vi "VS-Temp Calibration.vi"(0 "Scale":T1={"Slope"=0.0, "Offset"=0.0, "Limits"={"Min"=0.0, "Max"=0.0}, "term config"=-1} {"term config" items=["default"=-1, "RSE"=10083, "NRSE"=10078, "Differential"=10106, "Pseudodifferential"=12529]}) -> (4 "Cluster out":T1={"Slope"=0.0, "Offset"=0.0, "Limits"={"Min"=0.0, "Max"=0.0}, "term config"=-1} {"term config" items=["default"=-1, "RSE"=10083, "NRSE"=10078, "Differential"=10106, "Pseudodifferential"=12529]}, 8 "Canceled?":bool)   [LabVIEW 2020]
uses:
  Typedefs/PhysMon-Scale.ctl
  epl-vi-lib/Utility VIs/Array Manipulation VIs/Sort and Index (DBL).vi
  <vilib>/Analysis/NI_AALPro.lvlib
panel:
  out "Temp Offset In":dbl caption="Offset (deg C)"
  out "Temp Slope In":dbl caption="Scale (deg C/V)"
  in  "Temp Offset":dbl caption="Offset (deg C)"
  in  "Temp Slope":dbl caption="Scale (deg C/V)"
  in  "Fit line":bool
  out "Table":string[][](table)
  in  "Measure":bool
  in  "Temp (C)":dbl
  out "XY Graph":cluster{dbl[], dbl[]}[](graph)
  in  "Cancel":bool
  in  "OK":bool
  # "Previous"
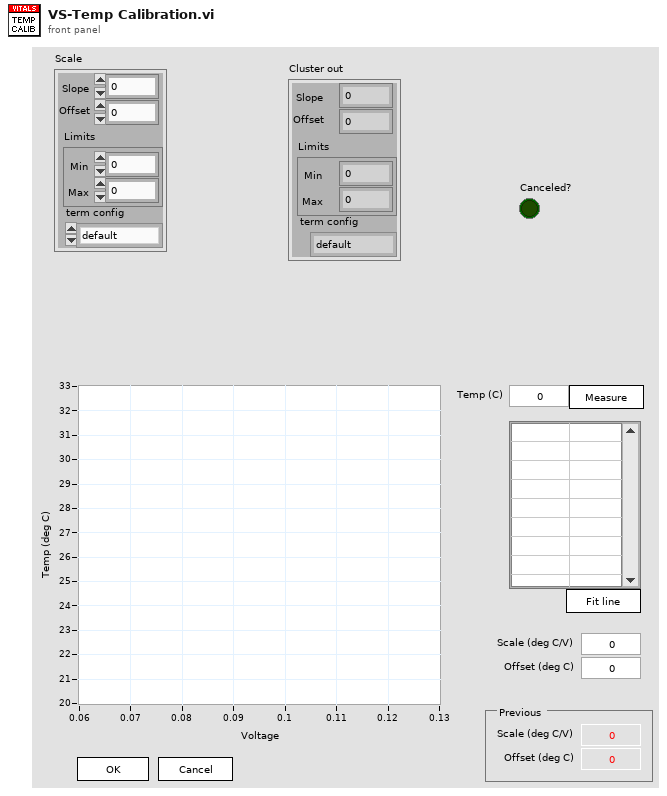
[diagram p1: front panel]
types:
  T1 = typedef "PhysMon-Scale.ctl" = cluster{"Slope":dbl, "Offset":dbl, "Limits":cluster{"Min":dbl, "Max":dbl}, "term config":i32}
  T2 = enum8{"Enabled", "Disabled", "Disabled and Grayed Out"}
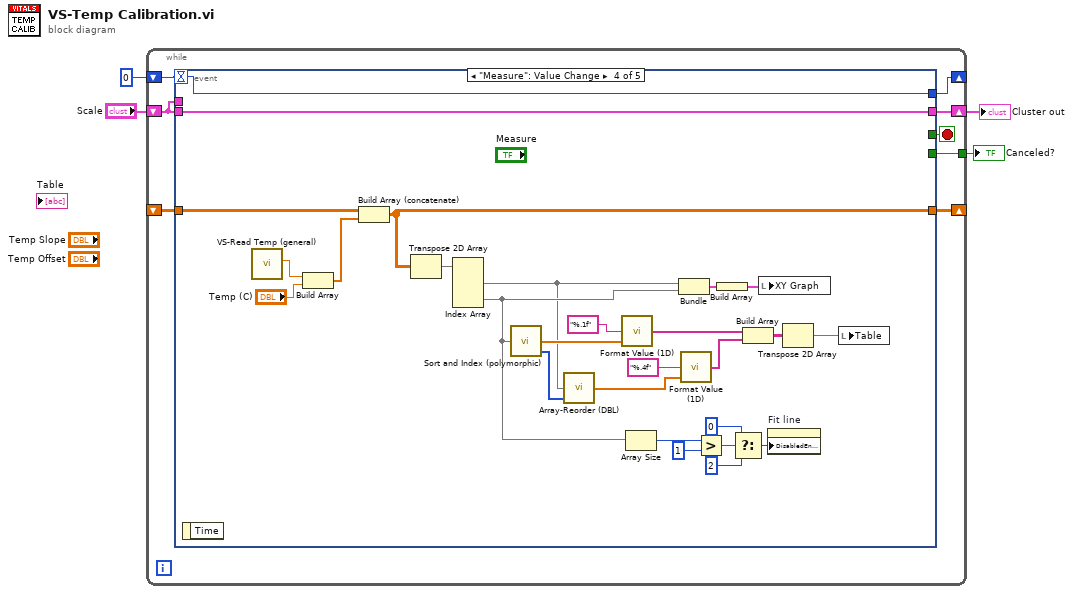
[diagram p0: block diagram]
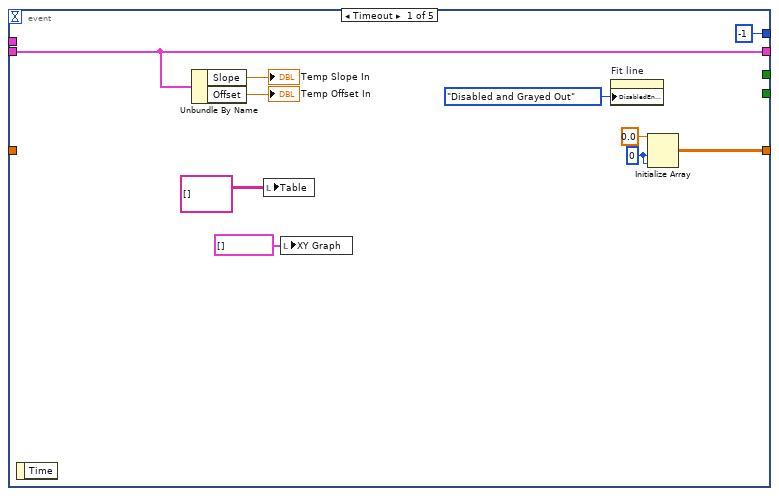
[diagram p2: hidden frame]
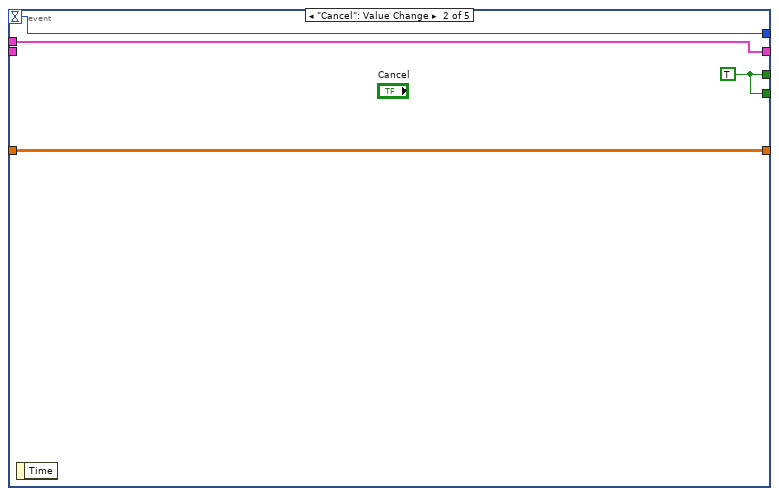
[diagram p3: hidden frame]
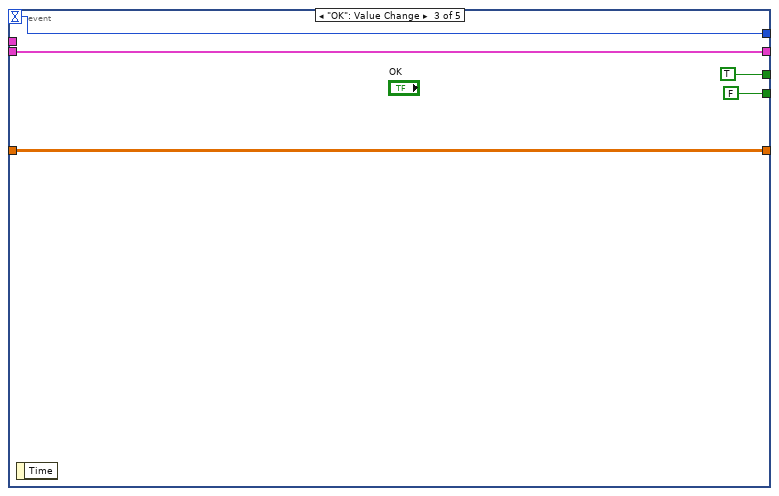
[diagram p4: hidden frame]
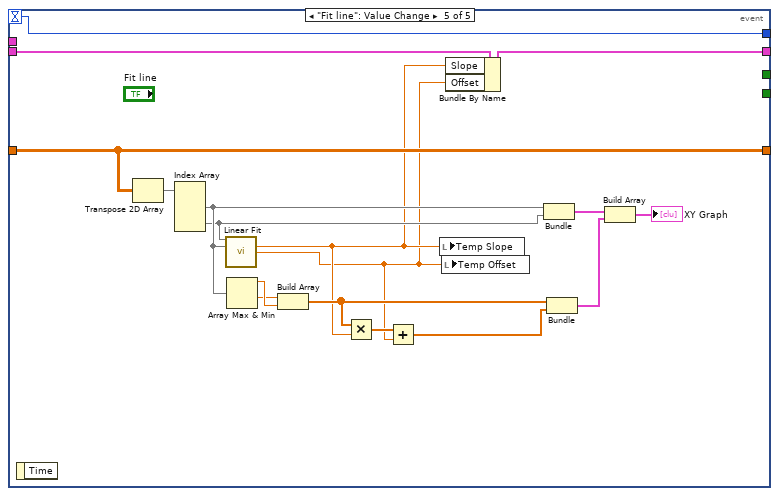
[diagram p5: hidden frame]
diagram:
  n1 = while {
    shift-right: [w11] -> _
    shift-left: 0 -> [w12]
    tunnel: [w8] -> w1
    shift-right: [w10] -> w2
    shift-left: "Scale" -> [w7]
    shift-right: [w6] -> _
    shift-left: _ -> [w5]
    stop <- w9 stop-if-true
    n2 = event shown="[3] \"Measure\": Value Change" {
      selector: _ -> [_ _ _ _ _]
      dyn-events: _ -> [_ _ _ _ _]
      timeout: w12 -> [_ w26 w30 w58 w75]
      tunnel: [-1 w26 w30 w58 w75] -> w11
      tunnel: w7 -> [w21 _ w31 w57 w74]
      tunnel: [w21 w24 w31 w57 w61] -> w10
      tunnel: [_ w25 TRUE _ _] -> w9
      tunnel: [_ w25 FALSE _ _] -> w8
      tunnel: w7 -> [_ w24 _ _ _]
      tunnel: [w16 w23 w27 w53 w73] -> w6
      tunnel: w5 -> [_ w23 w27 w56 w73]
      event Timeout {
        w15 = 0 ("dimension size")
        n3 = event-data() -> ()  [unwired: 1 in, 1 out]
        n4 = Unbundle By Name(w21) -> ("Slope"=→"Temp Slope In":dbl, "Offset"=→"Temp Offset In":dbl)
        n5 = local write "Table"(string[][] [] ("Table Control")) -> ()
        n6 = local write "XY Graph"(cluster{dbl[], dbl[]}[] [] ("XY Graph")) -> ()
        n7 = property on="Fit line" class="Bool"("DisabledEnum"=T2."Disabled and Grayed Out" ("Disabled")) -> ()  [unwired: 2 in, 2 out]
        n8 = Initialize Array(0.0 ("element"), w15, w15) -> (w16:dbl[][])
      }
      event "Cancel": Value Change {
        w25 = TRUE
        n9 = event-data() -> ()  [unwired: 1 in, 1 out]
      }
      event "OK": Value Change {
        n10 = event-data() -> ()  [unwired: 1 in, 1 out]
      }
      event "Measure": Value Change {
        n11 = event-data() -> ()  [unwired: 1 in, 1 out]
        n12 = call "VS-Read Temp (general).vi"() -> ("Vmean"=w32:dbl)  [unwired: 9 in, 2 out]
        n13 = Build Array(w32, "Temp (C)") -> (w55:dbl[])
        n14 = Build Array (concatenate)(w56, w55) -> (w53:dbl[][])
        n15 = Transpose 2D Array(2D array=w53) -> (transposed array=w54:dbl[][])
        n16 = Index Array(array=w54) -> (element #1=w37:dbl[], element #2=w39:dbl[])  [unwired: 4 in]
        n17 = call-poly "Sort and Index (polymorphic).vi"("X"=w39) -> ("Index"=w38:i32[], "Sort(X)"=w40:dbl[])  [unwired: 3 in]
        n18 = call "Array-Reorder (DBL).vi"("Index"=w38, "X"=w37) -> ("Reordered X"=w36:dbl[])  [unwired: 3 in]
        n19 = call "Format Value (1D).vi"("Array (DBL)"=w40, "format string"="%.1f") -> ("String Array"=w49:string[])  [unwired: 1 in]
        n20 = Array Size(array=w39) -> (size(s)=w46:i32)
        n21 = Bundle(w37, w39) -> (w34:cluster{dbl[], dbl[]})  [unwired: 1 in]
        n22 = call "Format Value (1D).vi"("Array (DBL)"=w36, "format string"="%.4f") -> ("String Array"=w50:string[])  [unwired: 1 in]
        n23 = Greater?(x=w46, y=1) -> (0:w44:bool)
        n24 = Build Array(w34) -> (w33:cluster{dbl[], dbl[]}[])
        n25 = Select(t=i16 0, s=w44, f=i16 2) -> (s? t:f=w43:i16)
        n26 = Build Array(w49, w50) -> (w48:string[][])
        n27 = local write "XY Graph"(w33) -> ()
        n28 = property on="Fit line" class="Bool"("DisabledEnum"=w43) -> ()  [unwired: 2 in, 2 out]
        n29 = Transpose 2D Array(2D array=w48) -> (transposed array=w47:string[][])
        n30 = local write "Table"(w47) -> ()
      }
      event "Fit line": Value Change {
        n31 = event-data() -> ()  [unwired: 1 in, 1 out]
        n32 = Transpose 2D Array(2D array=w73) -> (transposed array=w72:dbl[][])
        n33 = Index Array(array=w72) -> (element #1=w68:dbl[], element #2=w67:dbl[])  [unwired: 4 in]
        n34 = call <vilib>:"Linear Fit.vi"("Y"=w67, "X"=w68) -> ("slope"=w60:dbl, "intercept"=w59:dbl)  [unwired: 9 in, 3 out]
        n35 = Array Max & Min(array=w68) -> (max value=w71:dbl, min value=w70:dbl)  [unwired: 2 out]
        n36 = Build Array(w70, w71) -> (w66:dbl[])
        n37 = Multiply(x=w66, y=w60) -> (x*y=w69:dbl[])
        n38 = Add(x=w69, y=w59) -> (x+y=w65:dbl[])
        n39 = local write "Temp Slope"(w60) -> ()
        n40 = local write "Temp Offset"(w59) -> ()
        n41 = Bundle By Name(cluster=w74, "Slope"=w60, "Offset"=w59) -> (w61:T1)
        n42 = Bundle(w68, w67) -> (w64:cluster{dbl[], dbl[]})  [unwired: 1 in]
        n43 = Bundle(w66, w65) -> (w63:cluster{dbl[], dbl[]})  [unwired: 1 in]
        n44 = Build Array(w64, w63) -> (→"XY Graph":cluster{dbl[], dbl[]}[])
      }
    }
  }
  "Cluster out" <- w2
  "Canceled?" <- w1
